vi "Set Version Information.vi"(8 "error in (no error)":errorcluster, 11 "Test Executive Builder Model in":refnum<class "Test Executive Builder Model.lvclass">) -> (0 "error out":errorcluster, 3 "Test Executive Builder Model out":refnum<class "Test Executive Builder Model.lvclass">)   [LabVIEW 2017, in "Test Executive Builder Model.lvclass"]
uses:
  Test Executive Builder Model.lvclass
  <vilib>/gpm_packages/@cs/test-executive/Source/Test Executive/TestExecutive Ref/TestExecutive Ref.lvclass
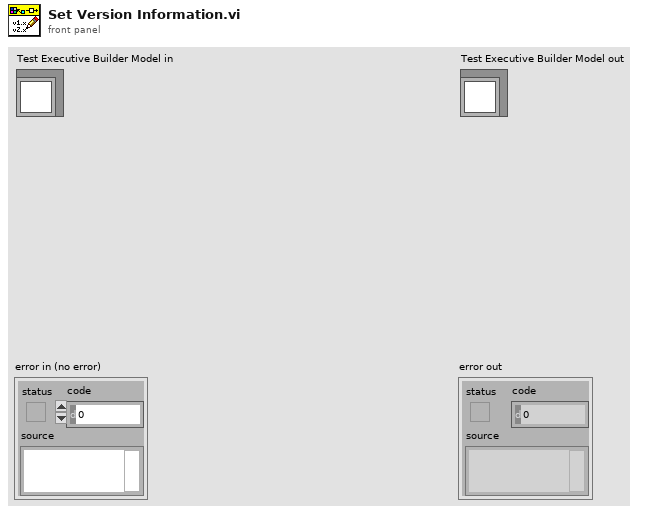
[diagram p1: front panel]
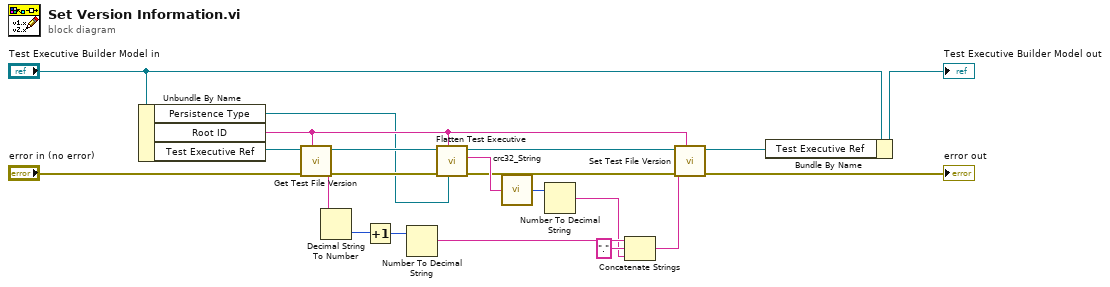
[diagram p0: block diagram]
diagram:
  n1 = Unbundle By Name("Test Executive Builder Model in") -> ("Persistence Type"=w5:refnum<class "IPersist.lvclass">, "Root ID"=w9:string, "Test Executive Ref"=w21:refnum<data-value>)
  n2 = call <vilib>:"Get Test File Version.vi"("Unique ID"=w9, "error in (no error)"="error in (no error)", "Test Executive Ref"=w21) -> ("error out"=w7:errorcluster, "Test File Version"=w15:string, "Test Executive Ref out"=w10:refnum<data-value>)  [unwired: 5 in, 1 out]
  n3 = Decimal String To Number(string=w15) -> (number=w14:i32)  [unwired: 2 in, 1 out]
  n4 = Increment(x=w14) -> (x+1=w13:i32)
  n5 = Number To Decimal String(number=w13) -> (decimal integer string=w12:string)  [unwired: 1 in]
  n6 = call <vilib>:"Flatten Test Executive.vi"("Persistence in"=w5, "Root ID"=w9, "error in (no error)"=w7, "Test Executive Ref"=w10) -> ("error out"=w6:errorcluster, "Flattened Test Executive"=w11:string, "Test Executive Ref out"=w8:refnum<data-value>)  [unwired: 5 in]
  n7 = call "crc32_String.vi"("String in"=w11) -> ("CRC32"=w2:u32)  [unwired: 1 in]
  n8 = Number To Decimal String(number=w2) -> (decimal integer string=w1:string)  [unwired: 1 in]
  n9 = Concatenate Strings(w12, "." ("string"), w1) -> (w4:string)
  n10 = call <vilib>:"Set Test File Version.vi"("Unique ID"=w9, "error in (no error)"=w6, "Test File Version"=w4, "Test Executive Ref"=w8) -> ("error out"=→"error out":errorcluster, "Test Executive Ref out"=w18:refnum<data-value>)  [unwired: 6 in]
  n11 = Bundle By Name(cluster="Test Executive Builder Model in", "Test Executive Ref"=w18) -> (→"Test Executive Builder Model out":refnum<class "Test Executive Builder Model.lvclass">)
